vi "read_serial_string.vi"(4 "serial read Buffer":string) -> (1 "unsigned long":u32)   [LabVIEW 2011]
doc: "Takes a unsigned long (4-byte) number that was send via the serial interface and transforms it into a unsigned long usable in labview. \n\nShould work with shorter numbers as well. Might only work with unsigned numbers???\n\nJohanens Rebling, 06/14/2012\nUofA"
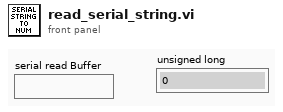
[diagram p1: front panel]
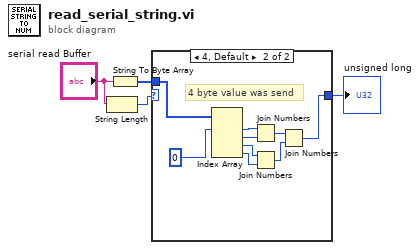
[diagram p0: block diagram]
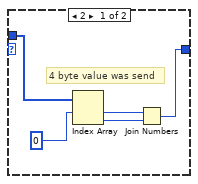
[diagram p2: hidden frame]
diagram:
  n1 = String Length(string="serial read Buffer") -> (length=w1:i32)
  n2 = String To Byte Array(string="serial read Buffer") -> (unsigned byte array=w4:u8[])
  n3 = case shown="4, Default" w1 {
    tunnel: w4 -> [w8 w10]
    tunnel: [w5 w11] -> w2
    frame 2 {
      # "4 byte value was send"
      n4 = Index Array(array=w8, index #1=0 ("index")) -> (element #1=w7:u8, element #2=w6:u8)  [unwired: 1 in]
      n5 = Join Numbers(hi=w7, lo=w6) -> ((hi.lo)=w5:u16)
    }
    frame 4, Default {
      # "4 byte value was send"
      n6 = Index Array(array=w10, index #1=0 ("index")) -> (element #1=w17:u8, element #2=w16:u8, element #3=w15:u8, element #4=w14:u8)  [unwired: 3 in]
      n7 = Join Numbers(hi=w17, lo=w16) -> ((hi.lo)=w13:u16)
      n8 = Join Numbers(hi=w15, lo=w14) -> ((hi.lo)=w12:u16)
      n9 = Join Numbers(hi=w13, lo=w12) -> ((hi.lo)=w11:u32)
    }
  }
  "unsigned long" <- w2
